vi "Create HTML.vi"(7 "FP Reference":refnum<class "Web Front Panel.lvclass">, 8 "error in (no error)":errorcluster, 10 "VI Identifier":string, 11 "String In":refnum<class "String.lvclass">) -> (0 "error out":errorcluster, 1 "js code for controls":string, 2 "js variables":string, 3 "String Out":refnum<class "String.lvclass">, 4 "script dependencies":string[](array[string]), 5 "HTML":string, 6 "js code for indicators":string)   [LabVIEW 2017, in "Front Panel Publisher.lvlib" / "String.lvclass"]
uses:
  String.lvclass
  Object_class/Object.lvclass
  Control_class/Control.lvclass
  Front Panel Publisher.lvlib
  Web Front Panel_class/Web Front Panel.lvclass
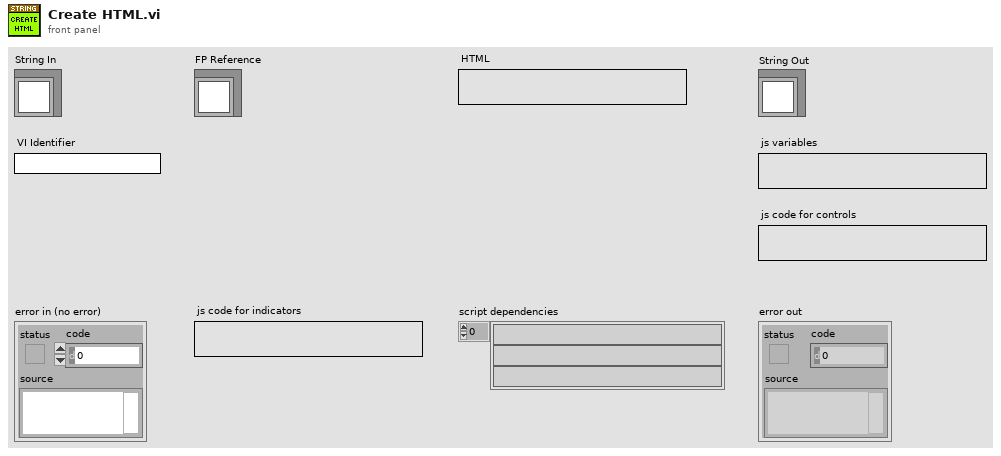
[diagram p1: front panel]
types:
  T1 = typedef "Front Panel Publisher.lvlib/Object.lvclass/Attributes.ctl" = cluster{"UID":i32, "Type":string, "Starting Location":T2, "Reference":refnum<vi>, "Cluster Component":bool, "Starting Rect Position":cluster{"Left":i16, "Top":i16}, "Owning Pane":refnum<vi>, "Master Total Rect Delta":T3}
  T2 = typedef "Front Panel Publisher.lvlib/Object.lvclass/Coordinates.ctl" = cluster{"Left":i32, "Top":i32, "Height":u32, "Width":u32}
  T3 = typedef "LVRectTypeDef.ctl" = cluster{"Left":i16, "Top":i16, "Right":i16, "Bottom":i16}
  T4 = typedef "Front Panel Publisher.lvlib/Control.lvclass/Attributes.ctl" = cluster{"Description":string, "Indicator":bool, "Default Value":variant, "Control Index":i32, "Label":refnum<class "Text.lvclass">, "Caption":refnum<class "Text.lvclass">, "Image b64":string, "No Control Index":bool, "Display Mode":T5}
  T5 = typedef "Front Panel Publisher.lvlib/Web Front Panel.lvclass/Enum - Control Display Mode.ctl" = enum16{"Value Only", "Value and Visibility", "Boolean Value Only", "Boolean Value and Visibility", "Control is Image", "Image and Visibility"}
  T6 = typedef "Front Panel Publisher.lvlib/String.lvclass/Attributes.ctl" = cluster{"String Is Path":bool}
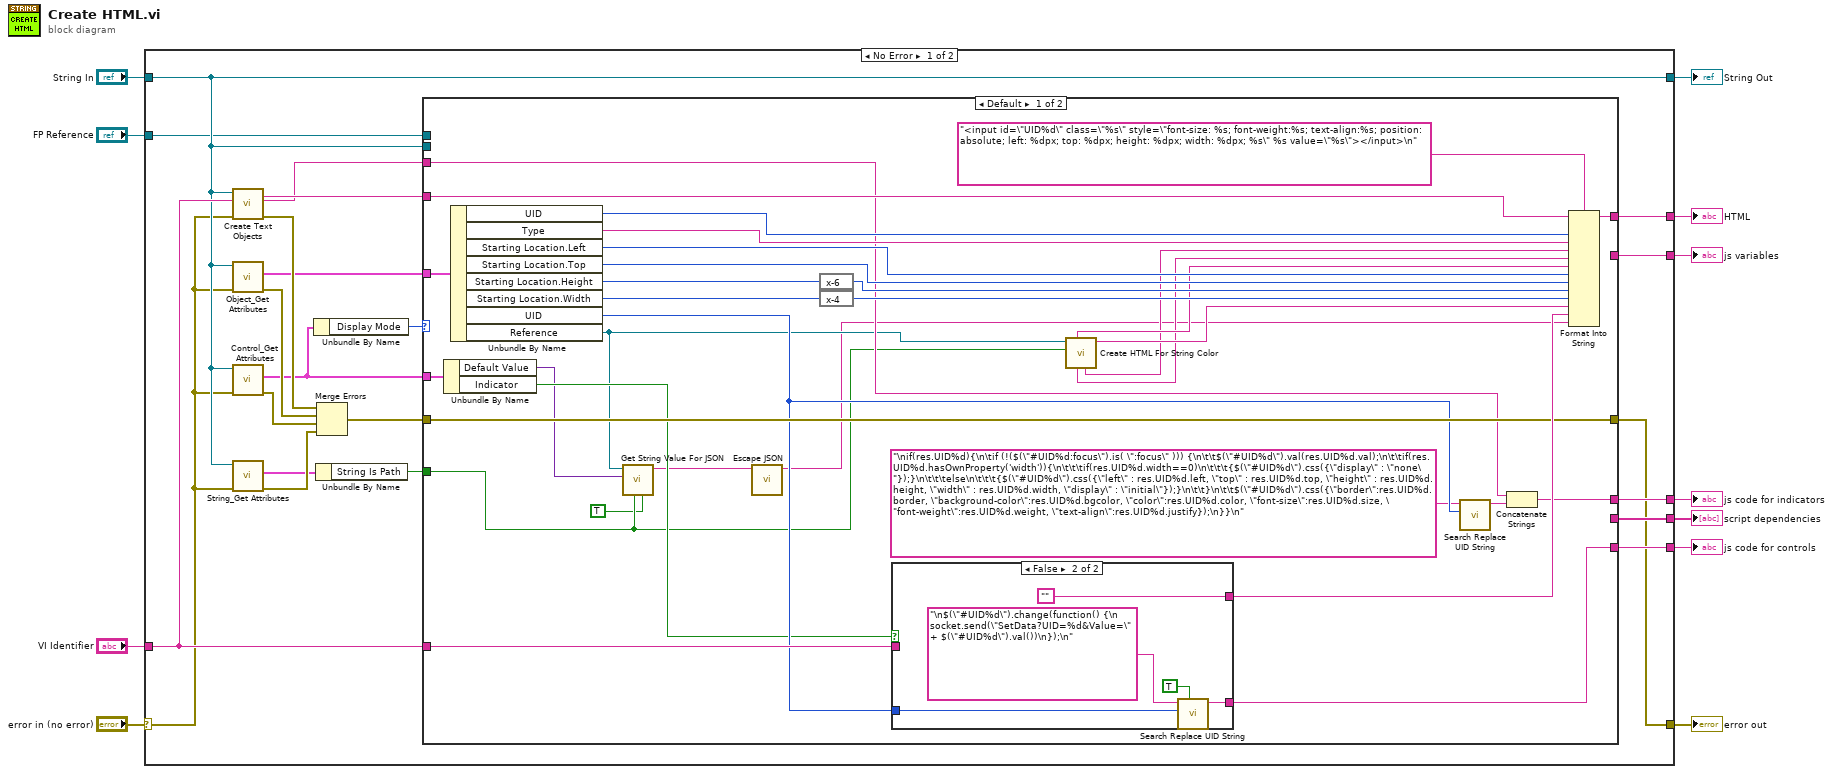
[diagram p0: block diagram]
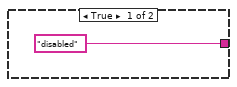
[diagram p2: hidden frame]
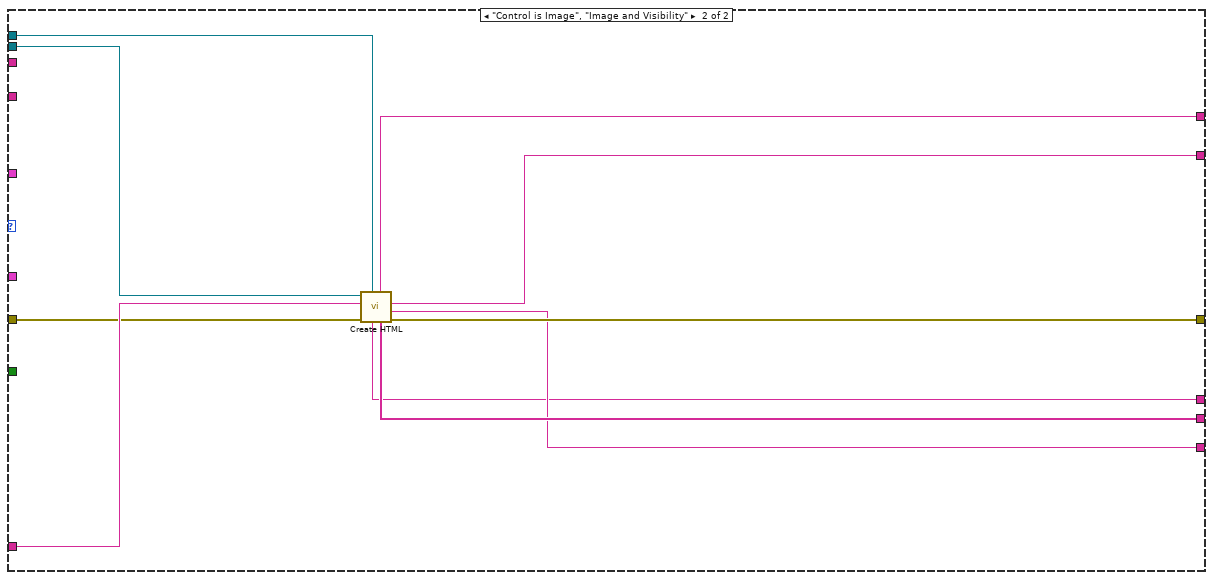
[diagram p3: hidden frame]
diagram:
  n1 = case shown="No Error" "error in (no error)" {
    selector: "error in (no error)" -> [w16 w84]
    tunnel: [w22 w84] -> w10
    tunnel: [w17 w83] -> w8
    tunnel: "String In" -> [w17 w83]
    tunnel: [w30 _] -> w7
    tunnel: [w28 _] -> w6
    tunnel: [w29 _] -> w5
    tunnel: "VI Identifier" -> [w26 _]
    tunnel: [w24 _] -> w3
    tunnel: [w23 _] -> w2
    tunnel: "FP Reference" -> [w12 _]
    frame No Error {
      n2 = call-dynamic "Create Text Objects.vi"("error in (no error)"=w16, "VI Name"=w26, "Control In"=w17) -> ("error out"=w31:errorcluster, "JS Indicator"=w19:string, "HTML"=w27:string)  [unwired: 5 in, 1 out]
      n3 = call "Object_Get Attributes.vi"("error in (no error)"=w16, "Object In"=w17) -> ("error out"=w32:errorcluster, "Object Attributes"=w18:T1)  [unwired: 7 in, 1 out]
      n4 = call "Control_Get Attributes.vi"("error in (no error)"=w16, "Control In"=w17) -> ("error out"=w33:errorcluster, "Control Attributes"=w21:T4)  [unwired: 7 in, 1 out]
      n5 = call "String_Get Attributes.vi"("error in (no error)"=w16, "String In"=w17) -> ("error out"=w15:errorcluster, "String Attributes"=w14:T6)  [unwired: 7 in, 1 out]
      n6 = Unbundle By Name(w21) -> ("Display Mode"=w20:T5)
      n7 = Unbundle By Name(w14) -> ("String Is Path"=w13:bool)
      n8 = Merge Errors(w31, w32, w33, w15) -> (w25:errorcluster)
      n9 = case shown="Default" w20 {
        tunnel: [w61 w77] -> w30
        tunnel: w18 -> [w46 _]
        tunnel: w21 -> [w56 _]
        tunnel: [w54 w75] -> w29
        tunnel: [w47 w74] -> w28
        tunnel: w27 -> [w53 _]
        tunnel: w26 -> [w52 w81]
        tunnel: w17 -> [_ w82]
        tunnel: w25 -> [w51 w80]
        tunnel: [_ w78] -> w24
        tunnel: [_ w76] -> w23
        tunnel: [w51 w79] -> w22
        tunnel: w19 -> [w45 _]
        tunnel: w13 -> [w38 _]
        tunnel: w12 -> [_ w73]
        frame Default {
          n10 = Unbundle By Name(w56) -> ("Default Value"=w39:variant, "Indicator"=w44:bool)
          n11 = Unbundle By Name(w46) -> ("UID"=w65:i32, "Type"=w64:string, "Starting Location.Left"=w63:i32, "Starting Location.Top"=w62:i32, "Starting Location.Height"=w60:u32, "Starting Location.Width"=w58:u32, "UID"=w49:i32, "Reference"=w37:refnum<vi>)
          n12 = call "Get String Value For JSON.vi"("No Control Index"=TRUE, "String Is Path"=w38, "Default Value"=w39, "GObject in"=w37) -> ("Text"=w35:string)  [unwired: 6 in, 1 out]
          n13 = call "Escape JSON.vi"("String in"=w35) -> ("String out"=w34:string)  [unwired: 10 in]
          n14 = expression code="x-6"(w60) -> (w59:u32)
          n15 = expression code="x-4"(w58) -> (w57:u32)
          n16 = case shown="False" w44 {
            tunnel: ["disabled" ""] -> w55
            tunnel: w49 -> [_ w70]
            tunnel: w52 -> [_ _]
            tunnel: [_ w69] -> w54
            frame True {
            }
            frame False {
              n17 = call "Search Replace UID String.vi"("Replace All Numeric Inputs"=TRUE, "UID"=w70, "Input String"="\n$(\"#UID%d\").change(function() {\n  socket.send(\"SetData?UID=%d&Value=\" + $(\"#UID%d\").val())\n});\n") -> ("Output String"=w69:string)  [unwired: 8 in]
            }
          }
          n18 = call "Create HTML For String Color.vi"("String Is Path"=w38, "GObject in"=w37) -> ("Style For Color"=w43:string, "Size"=w41:string, "Weight"=w40:string, "Justify"=w42:string)  [unwired: 2 in, 4 out]
          n19 = call "Search Replace UID String.vi"("UID"=w49, "Input String"="\nif(res.UID%d){\n\tif (!($(\"#UID%d:focus\").is( \":focus\" ))) {\n\t\t$(\"#UID%d\").val(res.UID%d.val);\n\t\tif(res.UID%d.hasOwnProperty('width')){\n\t\t\tif(res.UID%d.width==0)\n\t\t\t{$(\"#UID%d\").css({\"display\" : \"none\"});}\n\t\t\telse\n\t\t\t{$(\"#UID%d\").css({\"left\" : res.UID%d.left, \"top\" : res.UID%d.top, \"height\" : res.UID%d.height, \"width\" : res.UID%d.width, \"display\" : \"initial\"});}\n\t\t}\n\t\t$(\"#UID%d\").css({\"border\":res.UID%d.border, \"background-color\":res.UID%d.bgcolor, \"color\":res.UID%d.color, \"font-size\":res.UID%d.size, \"font-weight\":res.UID%d.weight, \"text-align\":res.UID%d.justify});\n}}\n") -> ("Output String"=w50:string)  [unwired: 9 in]
          n20 = Concatenate Strings(w45, w50) -> (w47:string)
          n21 = Format Into String(format string="<input id=\"UID%d\" class=\"%s\" style=\"font-size: %s; font-weight:%s; text-align:%s; position: absolute; left: %dpx; top: %dpx; height: %dpx; width: %dpx; %s\" %s value=\"%s\"></input>\n", initial string=w53, w65, w64, w41, w40, w42, w63, w62, w59, w57, w43, w55, w34) -> (resulting string=w61:string)  [unwired: 1 in, 1 out]
        }
        frame "Control is Image", "Image and Visibility" {
          n22 = call-parent "Create HTML.vi"("FP Reference"=w73, "error in (no error)"=w80, "VI Identifier"=w81, "Control In"=w82) -> ("error out"=w79:errorcluster, "js code for controls"=w75:string, "js variables"=w76:string, "script dependencies"=w78:string[], "HTML"=w77:string, "js code for indicators"=w74:string)  [unwired: 1 in, 1 out]
        }
      }
    }
    frame Error {
    }
  }
  "error out" <- w10
  "String Out" <- w8
  "HTML" <- w7
  "js variables" <- w2
  "js code for controls" <- w5
  "script dependencies" <- w3
  "js code for indicators" <- w6
